vi "Init.vi"(8 "Queue Mailbox":refnum<data-value>, 9 "Self Queue":refnum<data-value>, 10 "Self Queue Alias":string) -> (3 "Base Queue out":refnum<class "Base Queue.lvclass">)   [LabVIEW 2021, in "jettl.lvlib" / "Base Queue.lvlib" / "Base Queue.lvclass"]
uses:
  Base Queue.lvclass
  Base Queue.lvclass/Base Queue.ctl
  State/Nominal State/Nominal State.lvclass
  C:/git/jettl/jettl/jettl/Base Queue/State/State/State.lvclass
  Addresses/Addresses/Addresses.lvclass
  Msg Strategy/Msg Strategy.lvclass
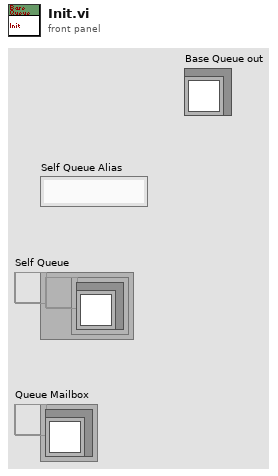
[diagram p1: front panel]
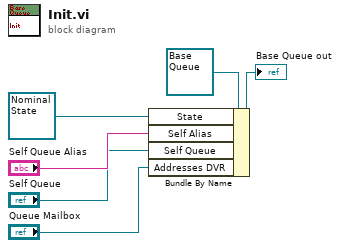
[diagram p0: block diagram]
diagram:
  n1 = Bundle By Name(cluster=refnum<class "Base Queue.lvclass"> refnum ("Self Actor in"), "State"=refnum<class "Nominal State.lvclass"> refnum ("jettl.lvlib:Nominal Queue State.lvclass"), "Self Alias"="Self Queue Alias", "Self Queue"="Self Queue", "Addresses DVR"="Queue Mailbox") -> (→"Base Queue out":refnum<class "Base Queue.lvclass">)
